vi "string array size.vi"(10 "array":string[](array[string])) -> (2 "size":u32)   [LabVIEW 2015]
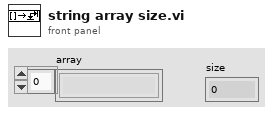
[diagram p1: front panel]
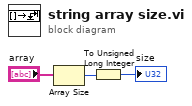
[diagram p0: block diagram]
diagram:
  n1 = Array Size(array="array") -> (size(s)=w3:i32)
  n2 = To Unsigned Long Integer(number=w3) -> (unsigned 32bit integer=→"size":u32)
